vi "Queue FGV.vi"(7 "Enum":enum16{"read", "write"}(ring), 11 "VI Communication In":T1) -> (3 "VI Communication Out":T1)   [LabVIEW 2024]
uses:
  state machine controller.ctl
  VI Communication.ctl
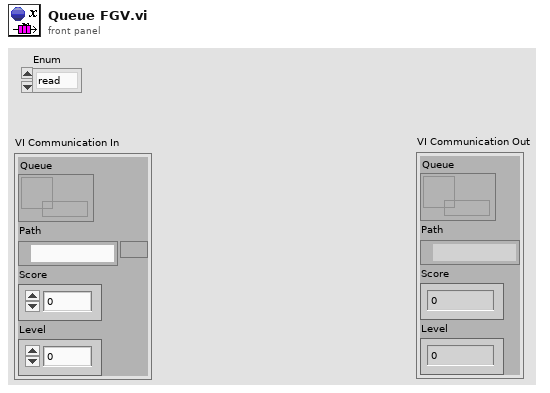
[diagram p1: front panel]
types:
  T1 = typedef "VI Communication.ctl" = cluster{"Queue":refnum<queue>, "Path":path, "Score":dbl, "Level":dbl}
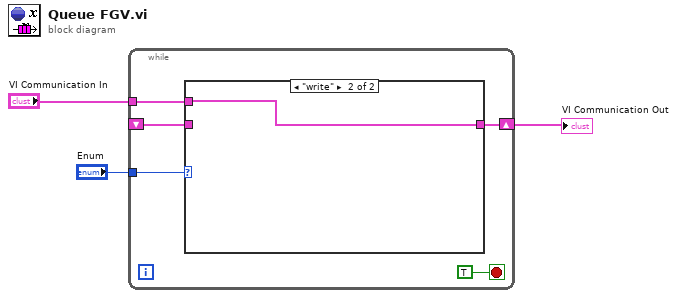
[diagram p0: block diagram]
diagram:
  n1 = while {
    tunnel: "Enum" -> [w8]
    shift-right: [w5] -> w1
    shift-left: _ -> [w7]
    tunnel: "VI Communication In" -> [w4]
    stop <- TRUE stop-if-true
    n2 = case shown="\"write\"" w8 {
      tunnel: w7 -> [w9 _]
      tunnel: [w9 w10] -> w5
      tunnel: w4 -> [_ w10]
      frame "read", Default {
      }
      frame "write" {
      }
    }
  }
  "VI Communication Out" <- w1
